vi "interp img path to lineout paths.vi"(8 "error in (no error)":errorcluster, 11 "Interp image path":path) -> (0 "error out":errorcluster, 2 "angle lineout path":path, 3 "Spectrum lineout path":path)   [LabVIEW 2020]
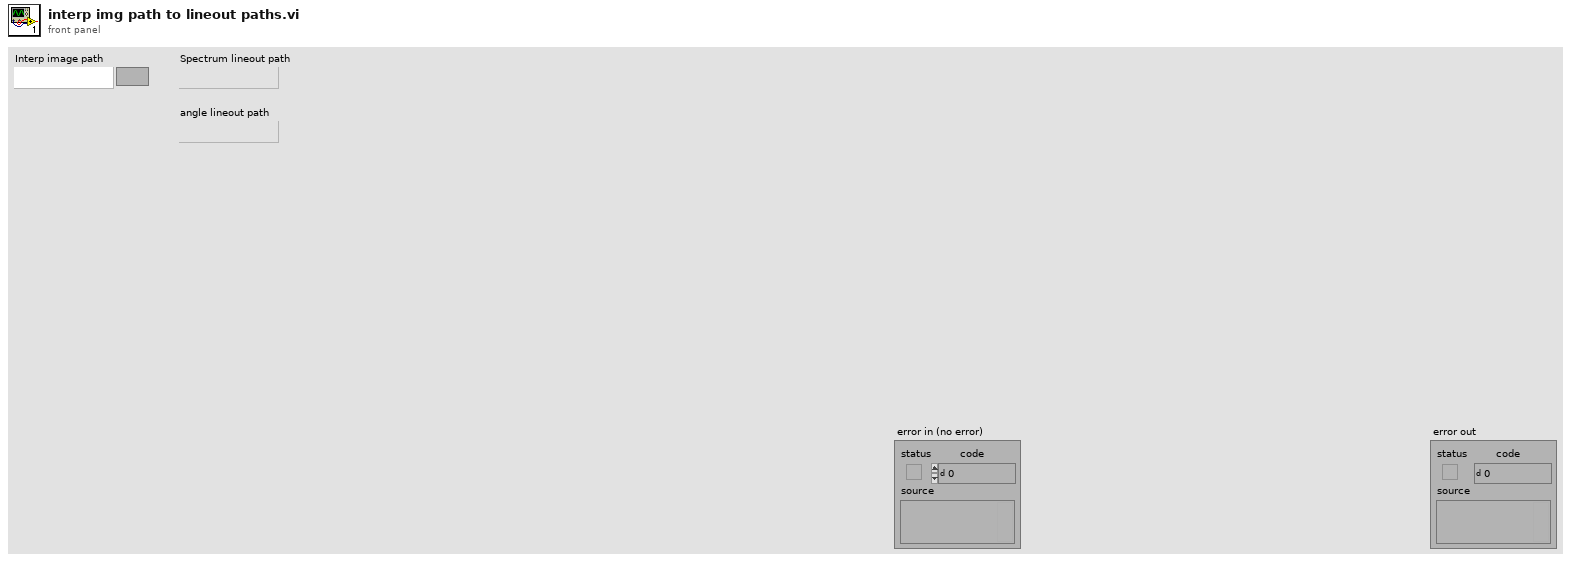
[diagram p1: front panel]
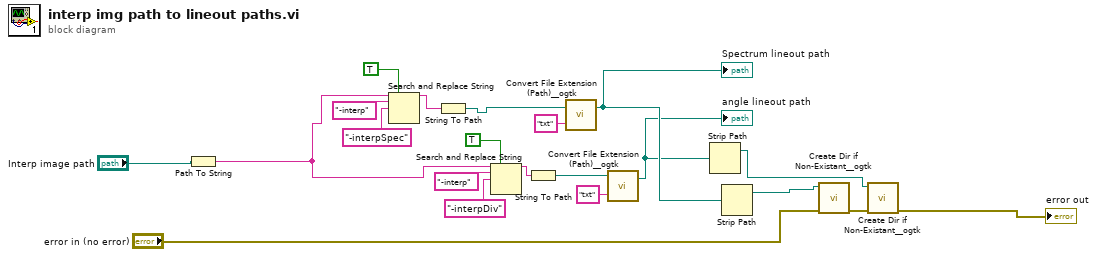
[diagram p0: block diagram]
diagram:
  n1 = Path To String(path="Interp image path") -> (string=w14:string)
  n2 = Search and Replace String(replace all?=TRUE ("replace all? (F)"), input string=w14, search string="-interp", replace string="-interpSpec") -> (result string=w12:string)  [unwired: 4 in, 3 out]
  n3 = String To Path(string=w12) -> (path=w9:path)
  n4 = Search and Replace String(replace all?=TRUE ("replace all? (F)"), input string=w14, search string="-interp", replace string="-interpDiv") -> (result string=w11:string)  [unwired: 4 in, 3 out]
  n5 = String To Path(string=w11) -> (path=w10:path)
  n6 = call "Convert File Extension (Path)__ogtk.vi"("new ending (none)"="txt", "file name"=w9) -> ("new filename"=w8:path)  [unwired: 1 out]
  "Spectrum lineout path" <- w8
  n7 = call "Convert File Extension (Path)__ogtk.vi"("new ending (none)"="txt", "file name"=w10) -> ("new filename"=w7:path)  [unwired: 1 out]
  "angle lineout path" <- w7
  n8 = Strip Path(path=w7) -> (stripped path=w5:path)  [unwired: 1 out]
  n9 = Strip Path(path=w8) -> (stripped path=w3:path)  [unwired: 1 out]
  n10 = call "Create Dir if Non-Existant__ogtk.vi"("error in (no error)"="error in (no error)", "Directory Path"=w3) -> ("error out"=w2:errorcluster)  [unwired: 7 in, 2 out]
  n11 = call "Create Dir if Non-Existant__ogtk.vi"("error in (no error)"=w2, "Directory Path"=w5) -> ("error out"=→"error out":errorcluster)  [unwired: 7 in, 2 out]
